vi "main.vi"() -> ()   [LabVIEW 2013]
uses:
  qwtblvlib/TD Quantity.ctl
  TD GUI Settings.ctl
  qwtblvlib/TD Backend Engine.ctl
  qwtblvlib/TD Algorithm Information.ctl
  qwtblvlib/TD Algorithm Information Input.ctl
  qwtblvlib/TD Algorithm Information Output.ctl
  qwtblvlib/TD Calculation Settings.ctl
  qwtblvlib/TD Uncertainty Calculation Method.ctl
  qwtblvlib/TD Correlation Calculation Settings.ctl
  qwtblvlib/TD DOF Calculation Settings.ctl
  qwtblvlib/TD MCM Calculation Settings.ctl
  qwtblvlib/TD MCM Calculation Method.ctl
  globals.vi
  <vilib>/Utility/xml.llb/Read From XML File(string).vi
  <vilib>/Utility/xml.llb/Write to XML File(string).vi
  qwtblvlib/QWTBLVLib.lvlib
panel:
  in  "show settings":bool
  in  "show algorithms":bool
  in  "show output data":bool
  in  "show input data":bool
  in  "calculate":bool
  in  "help":bool
  out "error out":errorcluster
  in  "quit":bool
  # "simple QWTB GUI"
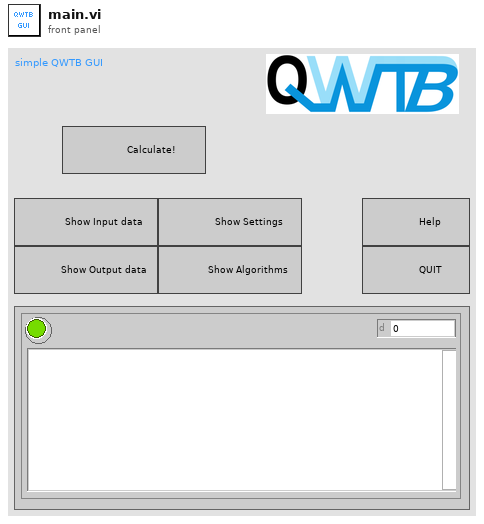
[diagram p1: front panel]
types:
  T1 = typedef "QWTBLVLib.lvlib/TD Quantity.ctl" = cluster{"Name":string, "Value":dbl[][], "Uncertainty":dbl[][], "Degrees of Freedom":dbl[][], "Correlation":dbl[][], "Randomized uncertainty":dbl[][]}
  T2 = typedef "QWTBLVLib.lvlib/TD Calculation Settings.ctl" = cluster{"Strict":bool, "Verbose":bool, "Uncertainty Calculation Method":T3, "Correlations":T4, "Degrees of Freedom":T5, "MCM Calculation Settings":T6}
  T3 = typedef "QWTBLVLib.lvlib/TD Uncertainty Calculation Method.ctl" = enum16{"none", "GUF", "MCM"}
  T4 = typedef "QWTBLVLib.lvlib/TD Correlation Calculation Settings.ctl" = cluster{"Required":bool, "Generate":bool}
  T5 = typedef "QWTBLVLib.lvlib/TD DOF Calculation Settings.ctl" = cluster{"Required":bool, "Generate":bool}
  T6 = typedef "QWTBLVLib.lvlib/TD MCM Calculation Settings.ctl" = cluster{"Repeats":i32, "Verbose":bool, "Parallelization method":T7, "Processors":i32, "Temporary directory":string, "Randomize":bool}
  T7 = typedef "QWTBLVLib.lvlib/TD MCM Calculation Method.ctl" = enum16{"Single Core", "Multi Core", "Multi Station"}
  T8 = typedef "QWTBLVLib.lvlib/TD Algorithm Information.ctl" = cluster{"ID":string, "Name":string, "Description":string, "Citation":string, "Remarks":string, "License":string, "Inputs":T9[], "Outputs":T10[], "Provides GUF":bool, "Provides MCM":bool, "Full path":string}
  T9 = typedef "QWTBLVLib.lvlib/TD Algorithm Information Input.ctl" = cluster{"Name":string, "Description":string, "Alternative":i32, "Optional":i32, "Parameter":i32}
  T10 = typedef "QWTBLVLib.lvlib/TD Algorithm Information Output.ctl" = cluster{"Name":string, "Description":string}
  T11 = typedef "TD GUI Settings.ctl" = cluster{"Backend engine":T12, "QWTB Folder Path":path}
  T12 = typedef "QWTBLVLib.lvlib/TD Backend Engine.ctl" = enum16{"Matlab by Script node", "GNU Octave by GOLPI"}
  T13 = enum32{"Invalid", "Standard", "Closed", "Hidden", "Minimized", "Maximized"}
  T14 = cluster{"Calculation Settings":T2, "GUI Settings":T11, "Data In":cluster{"Name":string, "Value":dbl[][], "Uncertainty":dbl[][], "Degrees of\nFreedom":dbl[][], "Correlation":dbl[][], "Randomized uncertainty":dbl[][]}[], "Available Algorithms":T8[], "Current Algorithm":T8, "Data Out":cluster{"Name":string, "Value":dbl[][], "Uncertainty":dbl[][], "Degrees of\nFreedom":dbl[][], "Correlation":dbl[][], "Randomized uncertainty":dbl[][]}[]}
  T15 = cluster{"Name":string, "Value":dbl[][], "Uncertainty":dbl[][], "Degrees of\nFreedom":dbl[][], "Correlation":dbl[][], "Randomized uncertainty":dbl[][]}[]
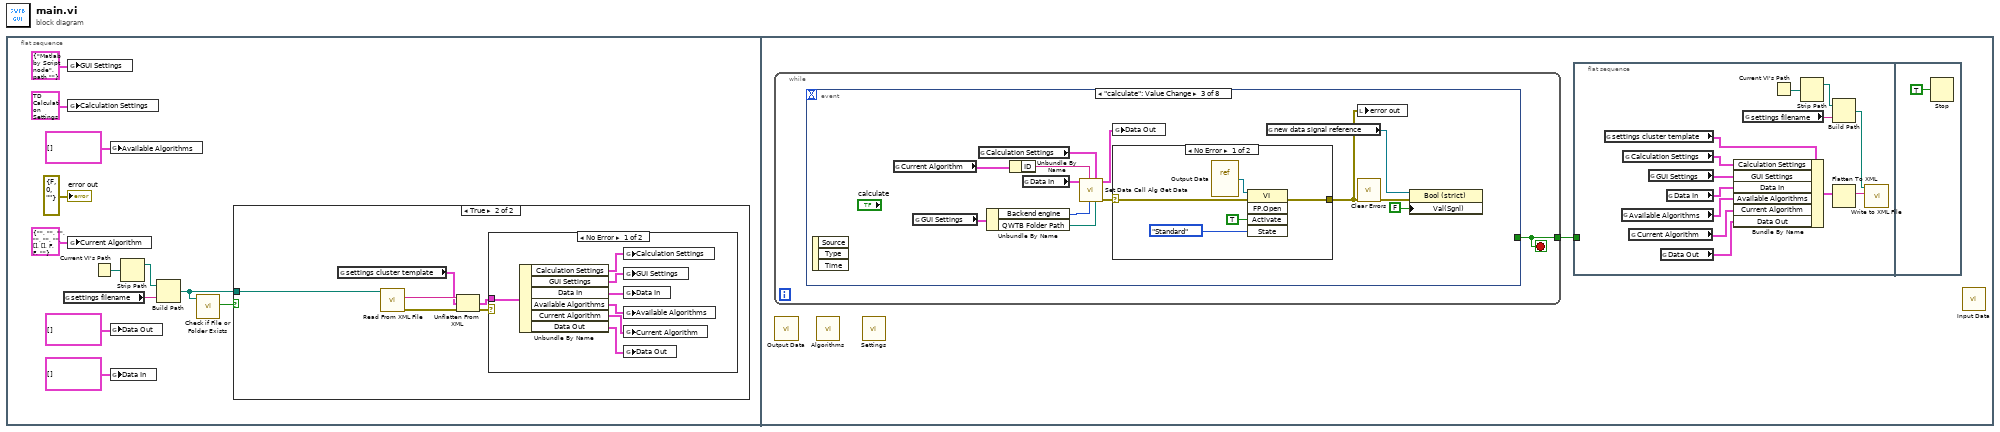
[diagram p0: block diagram]
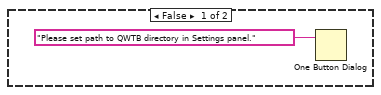
[diagram p2: hidden frame]
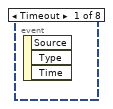
[diagram p4: hidden frame]
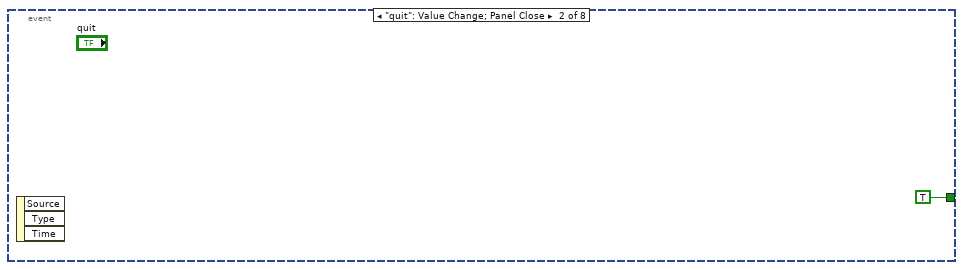
[diagram p5: hidden frame]
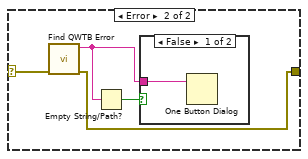
[diagram p6: hidden frame]
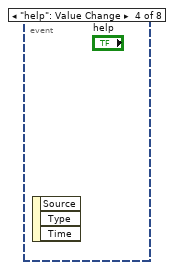
[diagram p8: hidden frame]
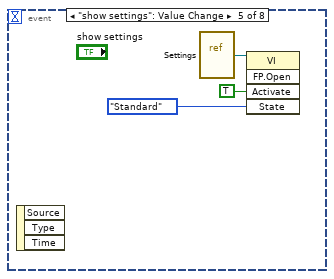
[diagram p9: hidden frame]
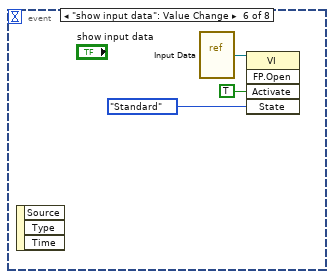
[diagram p10: hidden frame]
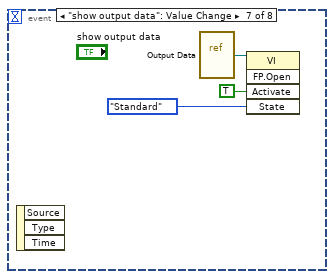
[diagram p11: hidden frame]
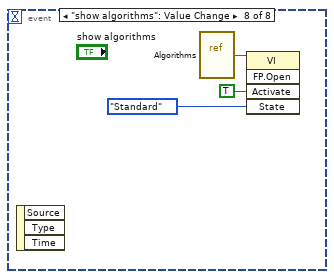
[diagram p12: hidden frame]
diagram:
  n1 = flat-sequence {
    frame #0 {
      n2 = global read "globals.vi" "settings filename"() -> (w7:string)
      n3 = global write "globals.vi" "GUI Settings"(T11 {"Backend engine"=enum."Matlab by Script node", "QWTB Folder Path"=path ""} ("GUI Settings")) -> ()
      n4 = global write "globals.vi" "Calculation Settings"(T2 {"Strict"=FALSE, "Verbose"=TRUE, "Uncertainty Calculation Method"=enum."none", "Correlations"={"Required"=FALSE, "Generate"=FALSE}, "Degrees of Freedom"={"Required"=FALSE, "Generate"=FALSE}, "MCM Calculation Settings"={"Repeats"=100, "Verbose"=TRUE, "Parallelization method"=enum."Single Core", "Processors"=0, "Temporary directory"=".", "Randomize"=TRUE}} ("Calculation Settings")) -> ()
      n5 = global write "globals.vi" "Current Algorithm"(T8 {"ID"="", "Name"="", "Description"="", "Citation"="", "Remarks"="", "License"="", "Inputs"=[], "Outputs"=[], "Provides GUF"=FALSE, "Provides MCM"=FALSE, "Full path"=""} ("Current Algorithm")) -> ()
      n6 = Current VI's Path() -> (path=w4:path)
      n7 = global write "globals.vi" "Available Algorithms"(T8[] [] ("Available Algorithms")) -> ()
      n8 = global write "globals.vi" "Data Out"(T1[] [] ("Data Out")) -> ()
      n9 = global write "globals.vi" "Data In"(T1[] []) -> ()
      n10 = Strip Path(path=w4) -> (stripped path=w3:path)  [unwired: 1 out]
      n11 = Build Path(base path=w3, name or relative path=w7) -> (appended path=w5:path)
      n12 = call <vilib>:"Check if File or Folder Exists.vi"("path"=w5) -> ("file or folder exists?"=w6:bool)  [unwired: 8 in, 2 out]
      n13 = case shown="True" w6 {
        tunnel: w5 -> [_ w15]
        frame False {
          n14 = One Button Dialog(message="Please set path to QWTB directory in Settings panel.") -> ()  [unwired: 1 in, 1 out]
        }
        frame True {
          n15 = global read "globals.vi" "settings cluster template"() -> (w14:T14)
          n16 = call-poly <vilib>:"Read From XML File.vi"("XML File Path"=w15) -> ("error out"=w18:errorcluster, "XML Elements"=w19:string)  [unwired: 8 in, 1 out]
          n17 = Unflatten From XML(xml string=w19, type=w14, error in (no error)=w18) -> (value=w16:T14, error out=w17:errorcluster)
          n18 = case shown="No Error" w17 {
            tunnel: w16 -> [w26 _]
            frame No Error {
              n19 = Unbundle By Name(w26) -> ("Calculation Settings"=w25:T2, "GUI Settings"=w24:T11, "Data In"=w23:T15, "Available Algorithms"=w22:T8[], "Current Algorithm"=w21:T8, "Data Out"=w20:T15)
              n20 = global write "globals.vi" "Calculation Settings"(w25) -> ()
              n21 = global write "globals.vi" "GUI Settings"(w24) -> ()
              n22 = global write "globals.vi" "Data In"(w23) -> ()
              n23 = global write "globals.vi" "Available Algorithms"(w22) -> ()
              n24 = global write "globals.vi" "Current Algorithm"(w21) -> ()
              n25 = global write "globals.vi" "Data Out"(w20) -> ()
            }
            frame Error {
            }
          }
        }
      }
      "error out" <- errorcluster {"status"=FALSE, "code"=0, "source"=""} ("error constant")
    }
    frame #1 {
      n26 = while {
        tunnel: [w42] -> w27
        stop <- w42 stop-if-true
        n27 = event shown="[2] \"calculate\": Value Change" {
          selector: _ -> [_ _ _ _ _ _ _ _]
          dyn-events: _ -> [_ _ _ _ _ _ _ _]
          timeout: _ -> [_ _ _ _ _ _ _ _]
          tunnel: [_ TRUE _ _ _ _ _ _] -> w42
          event Timeout {
            n28 = event-data() -> ()  [unwired: 1 in, 3 out]
          }
          event "quit": Value Change; Panel Close {
            n29 = event-data() -> ()  [unwired: 1 in, 3 out]
          }
          event "calculate": Value Change {
            n30 = event-data() -> ()  [unwired: 1 in, 3 out]
            n31 = global read "globals.vi" "Current Algorithm"() -> (w47:T8)
            n32 = global read "globals.vi" "GUI Settings"() -> (w51:T11)
            n33 = global read "globals.vi" "Calculation Settings"() -> (w52:T2)
            n34 = Unbundle By Name(w51) -> ("Backend engine"=w50:T12, "QWTB Folder Path"=w49:path)
            n35 = Unbundle By Name(w47) -> ("ID"=w46:string)
            n36 = global read "globals.vi" "Data In"() -> (w56:T15)
            n37 = call "Set Data Call Alg Get Data.vi"("QWTB Folder Path"=w49, "Calculation Settings"=w52, "Backend engine"=w50, "Algorithm ID"=w46, "Data In"=w56) -> ("error out"=w45:errorcluster, "Data Out"=w55:T1[])  [unwired: 5 in]
            n38 = global write "globals.vi" "Data Out"(w55) -> ()
            n39 = case shown="No Error" w45 {
              selector: w45 -> [w58 w65]
              tunnel: [w57 w64] -> w44
              frame No Error {
                n40 = vi-ref "Output Data.vi"() -> (w61:refnum<vi>)
                n41 = invoke class="VI" method="FP.Open"(reference=w61, error in=w58, "Activate"=TRUE ("Activate?"), "State"=T13."Standard") -> (error out=w57:errorcluster)  [unwired: 1 in, 4 out]
              }
              frame Error {
                n42 = call "Find QWTB Error.vi"("error in (no error)"=w65) -> ("error out"=w64:errorcluster, "QWTB error\n(empty string)"=w62:string)  [unwired: 8 in, 1 out]
                n43 = Empty String/Path?(string/path=w62) -> (empty?=w63:bool)
                n44 = case shown="False" w63 {
                  tunnel: w62 -> [w66 _]
                  frame False {
                    n45 = One Button Dialog(message=w66) -> ()  [unwired: 1 in, 1 out]
                  }
                  frame True {
                  }
                }
              }
            }
            n46 = global read "globals.vi" "new data signal reference"() -> (w54:refnum<vi>)
            n47 = local write "error out"(w44) -> ()
            n48 = call <vilib>:"Clear Errors.vi"("error in (no error)"=w44) -> ("error out"=w48:errorcluster)  [unwired: 6 in]
            n49 = property class="Bool (strict)"(reference=w54, error in=w48, "Val(Sgnl)"=FALSE ("Value (Signaling)")) -> ()  [unwired: 2 out]
          }
          event "help": Value Change {
            n50 = event-data() -> ()  [unwired: 1 in, 3 out]
          }
          event "show settings": Value Change {
            n51 = event-data() -> ()  [unwired: 1 in, 3 out]
            n52 = vi-ref "Settings.vi"() -> (w69:refnum<vi>)
            n53 = invoke class="VI" method="FP.Open"(reference=w69, "Activate"=TRUE ("Activate?"), "State"=T13."Standard") -> ()  [unwired: 2 in, 5 out]
          }
          event "show input data": Value Change {
            n54 = event-data() -> ()  [unwired: 1 in, 3 out]
            n55 = vi-ref "Input Data.vi"() -> (w72:refnum<vi>)
            n56 = invoke class="VI" method="FP.Open"(reference=w72, "Activate"=TRUE ("Activate?"), "State"=T13."Standard") -> ()  [unwired: 2 in, 5 out]
          }
          event "show output data": Value Change {
            n57 = event-data() -> ()  [unwired: 1 in, 3 out]
            n58 = vi-ref "Output Data.vi"() -> (w75:refnum<vi>)
            n59 = invoke class="VI" method="FP.Open"(reference=w75, "Activate"=TRUE ("Activate?"), "State"=T13."Standard") -> ()  [unwired: 2 in, 5 out]
          }
          event "show algorithms": Value Change {
            n60 = event-data() -> ()  [unwired: 1 in, 3 out]
            n61 = vi-ref "Algorithms.vi"() -> (w78:refnum<vi>)
            n62 = invoke class="VI" method="FP.Open"(reference=w78, "Activate"=TRUE ("Activate?"), "State"=T13."Standard") -> ()  [unwired: 2 in, 5 out]
          }
        }
      }
      n63 = call "Output Data.vi"() -> ()  [unwired: 12 in]
      n64 = call "Algorithms.vi"() -> ()  [unwired: 12 in]
      n65 = call "Settings.vi"() -> ()  [unwired: 12 in]
      n66 = flat-sequence {
        tunnel: w27 -> [_]
        frame #0 {
          n67 = global read "globals.vi" "settings cluster template"() -> (w33:T14)
          n68 = global read "globals.vi" "Available Algorithms"() -> (w37:T8[])
          n69 = global read "globals.vi" "Calculation Settings"() -> (w40:T2)
          n70 = global read "globals.vi" "Current Algorithm"() -> (w36:T8)
          n71 = global read "globals.vi" "GUI Settings"() -> (w39:T11)
          n72 = global read "globals.vi" "Data Out"() -> (w35:T15)
          n73 = global read "globals.vi" "Data In"() -> (w38:T15)
          n74 = Bundle By Name(cluster=w33, "Calculation Settings"=w40, "GUI Settings"=w39, "Data In"=w38, "Available Algorithms"=w37, "Current Algorithm"=w36, "Data Out"=w35) -> (w34:T14)
          n75 = global read "globals.vi" "settings filename"() -> (w31:string)
          n76 = Current VI's Path() -> (path=w29:path)
          n77 = Strip Path(path=w29) -> (stripped path=w28:path)  [unwired: 1 out]
          n78 = Build Path(base path=w28, name or relative path=w31) -> (appended path=w32:path)
          n79 = Flatten To XML(anything=w34) -> (xml string=w30:string)
          n80 = call-poly <vilib>:"Write to XML File.vi"("XML Input"=w30, "XML File Path"=w32) -> ()  [unwired: 7 in, 3 out]
        }
        frame #1 {
          n81 = Stop(stop? (T)=TRUE) -> ()
        }
      }
      n82 = call "Input Data.vi"() -> ()  [unwired: 12 in]
    }
  }
